vi "Delete Measurement Queue From Table.vi"(8 "error in (no error)":errorcluster, 10 "Unique Identifier":string, 11 "Controller in":refnum<class "Controller.lvclass">) -> (0 "error out":errorcluster, 3 "Controller out":refnum<class "Controller.lvclass">)   [LabVIEW 2015, in "Controller Actor.lvlib" / "Controller.lvclass"]
uses:
  Controller.lvclass
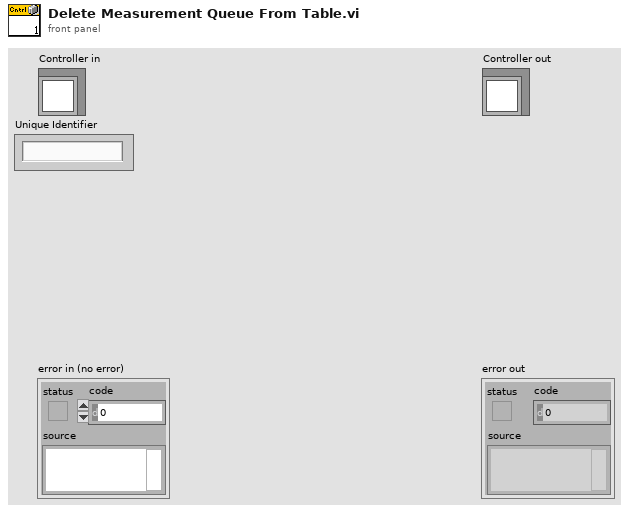
[diagram p1: front panel]
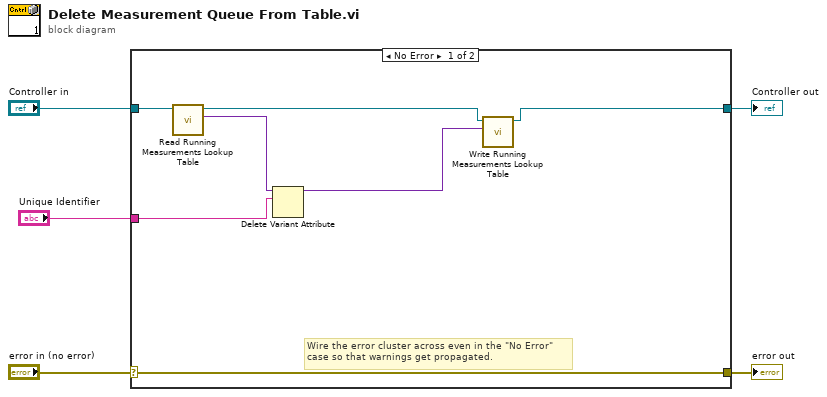
[diagram p0: block diagram]
diagram:
  n1 = case shown="No Error" "error in (no error)" {
    selector: "error in (no error)" -> [w12 w14]
    tunnel: [w12 w14] -> w4
    tunnel: [w6 w13] -> w2
    tunnel: "Controller in" -> [w8 w13]
    tunnel: "Unique Identifier" -> [w11 _]
    frame No Error {
      # "Wire the error cluster across even in the \"No Error\"\ncase so that warnings get propagated."
      n2 = call "Read Running Measurements Lookup Table.vi"("Controller in"=w8) -> ("Running Measurements Lookup Table"=w10:variant, "Controller out"=w7:refnum<class "Controller.lvclass">)  [unwired: 8 in, 1 out]
      n3 = Delete Variant Attribute(6:w11, 7:w10) -> (3:w9:variant)  [unwired: 1 in, 2 out]
      n4 = call "Write Running Measurements Lookup Table.vi"("Running Measurements Lookup Table"=w9, "Controller in"=w7) -> ("Controller out"=w6:refnum<class "Controller.lvclass">)  [unwired: 8 in, 1 out]
    }
    frame Error {
    }
  }
  "error out" <- w4
  "Controller out" <- w2
